vi "Main_ProductionMonitor.vi"() -> ()   [LabVIEW 2017]
uses:
  ScanPLC_Config.vi
panel:
  out "LineName":string
  in  "Cluster":cluster{"Goal":dbl}
  out "Shift":string
  out "Date/Time":string
  in  "stop":bool
  in  "Tab":T1(tab)
  out "PLC Count Int":i32
  out "PLC Count Bool":bool
  in  "ProductionToCloud":bool
  out "ProductionBoard":T2={"StartHour"=[{"Hour"=5, "Minute"=0}, {"Hour"=6, "Minute"=0}, {"Hour"=7, "Minute"=0}, {"Hour"=7, "Minute"=30}, {"Hour"=0, "Minute"=0}, {"Hour"=0, "Minute"=0}, {"Hour"=0, "Minute"=0}, {"Hour"=0, "Minute"=0}, {"Hour"=0, "Minute"=0}], "Goal"=[], "EndHour"=[{"Hour"=5, "Minute"=59}, {"Hour"=6, "Minute"=59}, {"Hour"=7, "Minute"=10}, {"Hour"=7, "Minute"=59}, {"Hour"=0, "Minute"=0}, {"Hour"=0, "Minute"=0}, {"Hour"=0, "Minute"=0}, {"Hour"=0, "Minute"=0}, {"Hour"=0, "Minute"=0}], "AM/PM"=[{"AM/PM"=0}, {"AM/PM"=0}, {"AM/PM"=0}, {"AM/PM"=0}, {"AM/PM"=0}, {"AM/PM"=0}, {"AM/PM"=0}, {"AM/PM"=0}, {"AM/PM"=0}], "Actual"=[], "%"=[], "Status"=[], "Comments"=[]} {"AM/PM"."AM/PM" items=["AM", "PM"]; "EndHour"."Minute" items=["00", "1", "2", "3", "4", "5", "6", "7", "8", "9", "10", "11", "12", "13", "14", "15", "16", "17", "18", "19", "20", "21", "22", "23", "24", "25", "26", "27", "28", "29", "30", "31", "32", "33", "34", "35", "36", "37", "38", "39", "40", "41", "42", "43", "44", "45", "46", "47", "48", "49", "50", "51", "52", "53", "54", "55", "56", "57", "58", "59"]; "EndHour"."Hour" items=["00", "1", "2", "3", "4", "5", "6", "7", "8", "9", "10", "11", "12", "13", "14", "15", "16", "17", "18", "19", "20", "21", "22", "23"]; "StartHour"."Minute" items=["00", "1", "2", "3", "4", "5", "6", "7", "8", "9", "10", "11", "12", "13", "14", "15", "16", "17", "18", "19", "20", "21", "22", "23", "24", "25", "26", "27", "28", "29", "30", "31", "32", "33", "34", "35", "36", "37", "38", "39", "40", "41", "42", "43", "44", "45", "46", "47", "48", "49", "50", "51", "52", "53", "54", "55", "56", "57", "58", "59"]; "StartHour"."Hour" items=["00", "1", "2", "3", "4", "5", "6", "7", "8", "9", "10", "11", "12", "13", "14", "15", "16", "17", "18", "19", "20", "21", "22", "23"]}
  in  "ShiftsFromCloud":bool
  in  "ShiftsToCloud":bool
  in  "Refresh Button":bool
  in  "GoalCalc":bool
  in  "SaveShifts":bool
  in  "3rdShiftConfig":T3={"StartHour"=[{"Hour"=5, "Minute"=0}, {"Hour"=6, "Minute"=0}, {"Hour"=7, "Minute"=0}, {"Hour"=7, "Minute"=30}, {"Hour"=0, "Minute"=0}, {"Hour"=0, "Minute"=0}, {"Hour"=0, "Minute"=0}, {"Hour"=0, "Minute"=0}, {"Hour"=0, "Minute"=0}], "Goal"=[], "EndHour"=[{"Hour"=5, "Minute"=59}, {"Hour"=6, "Minute"=59}, {"Hour"=7, "Minute"=10}, {"Hour"=7, "Minute"=59}, {"Hour"=0, "Minute"=0}, {"Hour"=0, "Minute"=0}, {"Hour"=0, "Minute"=0}, {"Hour"=0, "Minute"=0}, {"Hour"=0, "Minute"=0}], "AM/PM"=[]} caption="3rdShift" {"AM/PM"."AM/PM" items=["AM", "PM"]; "EndHour"."Minute" items=["00", "1", "2", "3", "4", "5", "6", "7", "8", "9", "10", "11", "12", "13", "14", "15", "16", "17", "18", "19", "20", "21", "22", "23", "24", "25", "26", "27", "28", "29", "30", "31", "32", "33", "34", "35", "36", "37", "38", "39", "40", "41", "42", "43", "44", "45", "46", "47", "48", "49", "50", "51", "52", "53", "54", "55", "56", "57", "58", "59"]; "EndHour"."Hour" items=["0", "1", "2", "3", "4", "5", "6", "7", "8", "9", "10", "11", "12", "13", "14", "15", "16", "17", "18", "19", "20", "21", "22", "23"]; "StartHour"."Minute" items=["00", "1", "2", "3", "4", "5", "6", "7", "8", "9", "10", "11", "12", "13", "14", "15", "16", "17", "18", "19", "20", "21", "22", "23", "24", "25", "26", "27", "28", "29", "30", "31", "32", "33", "34", "35", "36", "37", "38", "39", "40", "41", "42", "43", "44", "45", "46", "47", "48", "49", "50", "51", "52", "53", "54", "55", "56", "57", "58", "59"]; "StartHour"."Hour" items=["0", "1", "2", "3", "4", "5", "6", "7", "8", "9", "10", "11", "12", "13", "14", "15", "16", "17", "18", "19", "20", "21", "22", "23"]}
  in  "2ndShiftConfig":T3={"StartHour"=[{"Hour"=5, "Minute"=0}, {"Hour"=6, "Minute"=0}, {"Hour"=7, "Minute"=0}, {"Hour"=7, "Minute"=30}, {"Hour"=0, "Minute"=0}, {"Hour"=0, "Minute"=0}, {"Hour"=0, "Minute"=0}, {"Hour"=0, "Minute"=0}, {"Hour"=0, "Minute"=0}], "Goal"=[], "EndHour"=[{"Hour"=5, "Minute"=59}, {"Hour"=6, "Minute"=59}, {"Hour"=7, "Minute"=10}, {"Hour"=7, "Minute"=59}, {"Hour"=0, "Minute"=0}, {"Hour"=0, "Minute"=0}, {"Hour"=0, "Minute"=0}, {"Hour"=0, "Minute"=0}, {"Hour"=0, "Minute"=0}], "AM/PM"=[{"AM/PM"=1}, {"AM/PM"=1}, {"AM/PM"=1}, {"AM/PM"=1}, {"AM/PM"=1}, {"AM/PM"=1}, {"AM/PM"=1}, {"AM/PM"=1}, {"AM/PM"=1}]} caption="2ndShift" {"AM/PM"."AM/PM" items=["AM", "PM"]; "EndHour"."Minute" items=["00", "1", "2", "3", "4", "5", "6", "7", "8", "9", "10", "11", "12", "13", "14", "15", "16", "17", "18", "19", "20", "21", "22", "23", "24", "25", "26", "27", "28", "29", "30", "31", "32", "33", "34", "35", "36", "37", "38", "39", "40", "41", "42", "43", "44", "45", "46", "47", "48", "49", "50", "51", "52", "53", "54", "55", "56", "57", "58", "59"]; "EndHour"."Hour" items=["00", "1", "2", "3", "4", "5", "6", "7", "8", "9", "10", "11", "12", "13", "14", "15", "16", "17", "18", "19", "20", "21", "22", "23"]; "StartHour"."Minute" items=["00", "1", "2", "3", "4", "5", "6", "7", "8", "9", "10", "11", "12", "13", "14", "15", "16", "17", "18", "19", "20", "21", "22", "23", "24", "25", "26", "27", "28", "29", "30", "31", "32", "33", "34", "35", "36", "37", "38", "39", "40", "41", "42", "43", "44", "45", "46", "47", "48", "49", "50", "51", "52", "53", "54", "55", "56", "57", "58", "59"]; "StartHour"."Hour" items=["0", "1", "2", "3", "4", "5", "6", "7", "8", "9", "10", "11", "12", "13", "14", "15", "16", "17", "18", "19", "20", "21", "22", "23"]}
  in  "1stShiftConfig":T3={"StartHour"=[{"Hour"=5, "Minute"=0}, {"Hour"=6, "Minute"=0}, {"Hour"=7, "Minute"=0}, {"Hour"=7, "Minute"=30}, {"Hour"=0, "Minute"=0}, {"Hour"=0, "Minute"=0}, {"Hour"=0, "Minute"=0}, {"Hour"=0, "Minute"=0}, {"Hour"=0, "Minute"=0}], "Goal"=[], "EndHour"=[{"Hour"=5, "Minute"=59}, {"Hour"=6, "Minute"=59}, {"Hour"=7, "Minute"=10}, {"Hour"=7, "Minute"=59}, {"Hour"=0, "Minute"=0}, {"Hour"=0, "Minute"=0}, {"Hour"=0, "Minute"=0}, {"Hour"=0, "Minute"=0}, {"Hour"=0, "Minute"=0}], "AM/PM"=[{"AM/PM"=0}, {"AM/PM"=0}, {"AM/PM"=0}, {"AM/PM"=0}, {"AM/PM"=0}, {"AM/PM"=0}, {"AM/PM"=0}, {"AM/PM"=0}, {"AM/PM"=0}]} caption="1stShift" {"AM/PM"."AM/PM" items=["AM", "PM"]; "EndHour"."Minute" items=["00", "1", "2", "3", "4", "5", "6", "7", "8", "9", "10", "11", "12", "13", "14", "15", "16", "17", "18", "19", "20", "21", "22", "23", "24", "25", "26", "27", "28", "29", "30", "31", "32", "33", "34", "35", "36", "37", "38", "39", "40", "41", "42", "43", "44", "45", "46", "47", "48", "49", "50", "51", "52", "53", "54", "55", "56", "57", "58", "59"]; "EndHour"."Hour" items=["0", "1", "2", "3", "4", "5", "6", "7", "8", "9", "10", "11", "12", "13", "14", "15", "16", "17", "18", "19", "20", "21", "22", "23"]; "StartHour"."Minute" items=["00", "1", "2", "3", "4", "5", "6", "7", "8", "9", "10", "11", "12", "13", "14", "15", "16", "17", "18", "19", "20", "21", "22", "23", "24", "25", "26", "27", "28", "29", "30", "31", "32", "33", "34", "35", "36", "37", "38", "39", "40", "41", "42", "43", "44", "45", "46", "47", "48", "49", "50", "51", "52", "53", "54", "55", "56", "57", "58", "59"]; "StartHour"."Hour" items=["0", "1", "2", "3", "4", "5", "6", "7", "8", "9", "10", "11", "12", "13", "14", "15", "16", "17", "18", "19", "20", "21", "22", "23"]}
  out "Parts/Hour":dbl
  in  "Cycle Time (s)":dbl=25.0
  in  "ShiftConfigPath":path
  in  "MainConfigFromCloud":bool
  in  "MainConfigBackup":bool
  in  "MainConfigPath":path
  in  "MainConfigurationArray":cluster{"Parameter":string, "Value":string}[](array[cluster])
  in  "SaveMailConfig":bool
  in  "RefreshMailConfig":bool
  out "NotificationMessage":string
  in  "Mail Button":bool
  in  "MainConfigToCloud":bool
  in  "PLC Connection Array":T4(array[cluster]) {"MemoryType" items=["CR (Control Relay)", "MR (Internal Auxiliary Relay)", "VB (Work Relay)", "LR (Latch Relay)", "B (Link Relay)", "R (Relay)", "DM (Data Memory)", "EM (Extended Data Memory)", "FM (File Register 1)", "ZF (FIle Register 2)", "W (Link Register)", "TM (Temporary Data Memory)", "Z (Index Register)", "T (Timer)", "TC (Timer (Counter Value))", "TS (Timer Set Value)", "C (Counter)", "CC (Counter (Counter Value))", "CS (Counter (Set Value))", "CTH (High Speed Counter)", "CTC (High Speed Counter Comparator (Set Value))", "AT (Digital Trimmer)", "CM (Control Memory)", "VM (Work Memory)"]; "PLC Type" items=["Keyence", "Allen Bradley", "Mitsubishi", "Panasonic", "Siemens"]}
  in  "PLCConfigPath":path
  in  "RefreshPLCConfig":bool
  in  "SavePLCConfig":bool
  # "Hourly Production Report"
  # "MachineName"
  # "PLC Address"
  # "PLC Type"
  # "Memory Type"
  # "MemoryNumber"
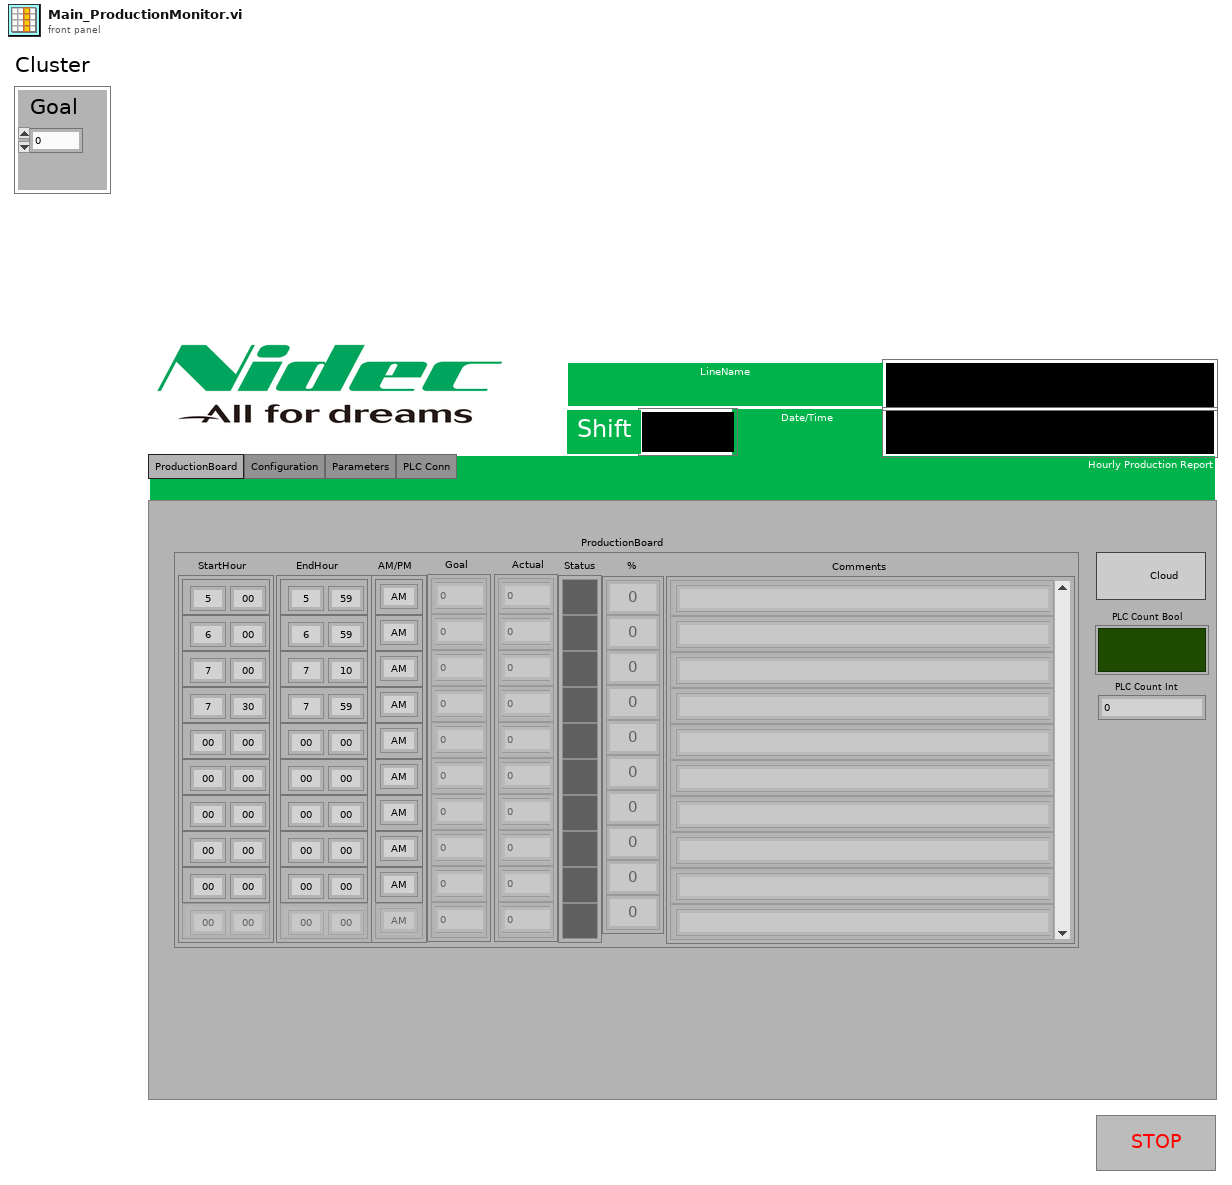
[diagram p1: front panel]
types:
  T1 = enum32{"ProductionBoard", "Configuration", "Parameters", "PLC Conn"}
  T2 = cluster{"StartHour":cluster{"Hour":u16, "Minute":u16}[], "Goal":cluster{"Goal":dbl}[], "EndHour":cluster{"Hour":u16, "Minute":u16}[], "AM/PM":cluster{"AM/PM":u16}[], "Actual":cluster{"Actual":dbl}[], "%":i32[], "Status":u32[], "Comments":cluster{"Comments":string}[]}
  T3 = cluster{"StartHour":cluster{"Hour":u16, "Minute":u16}[], "Goal":cluster{"Goal":dbl}[], "EndHour":cluster{"Hour":u16, "Minute":u16}[], "AM/PM":cluster{"AM/PM":u16}[]}
  T4 = cluster{"MachineName":string, "PLC Address":string, "PLC Type":u16, "MemoryType":u16, "MemoryNumber":i32}[]
  T5 = cluster{"MachineName":string, "PLC Address":string, "PLC Type":u16, "MemoryType":u16, "MemoryNumber":i32}
  T6 = cluster{"1stShiftConfig":cluster{"StartHour":cluster{"Hour":u16, "Minute":u16}[], "Goal":cluster{"Goal":dbl}[], "EndHour":cluster{"Hour":u16, "Minute":u16}[], "AM/PM":cluster{"AM/PM":u16}[]}, "2ndShiftConfig":cluster{"StartHour":cluster{"Hour":u16, "Minute":u16}[], "Goal":cluster{"Goal":dbl}[], "EndHour":cluster{"Hour":u16, "Minute":u16}[], "AM/PM":cluster{"AM/PM":u16}[]}, "3rdShiftConfig":cluster{"StartHour":cluster{"Hour":u16, "Minute":u16}[], "Goal":cluster{"Goal":dbl}[], "EndHour":cluster{"Hour":u16, "Minute":u16}[], "AM/PM":cluster{"AM/PM":u16}[]}}
  T7 = cluster{"Hour":cluster{"Hour":u16, "Minute":u16}}[]
  T8 = cluster{"InitialHour":u16, "InitialMinute":u16, "EndHour":u16, "EndMinute":u16, "Goal":dbl, "Actual":dbl, "Comments":string}[]
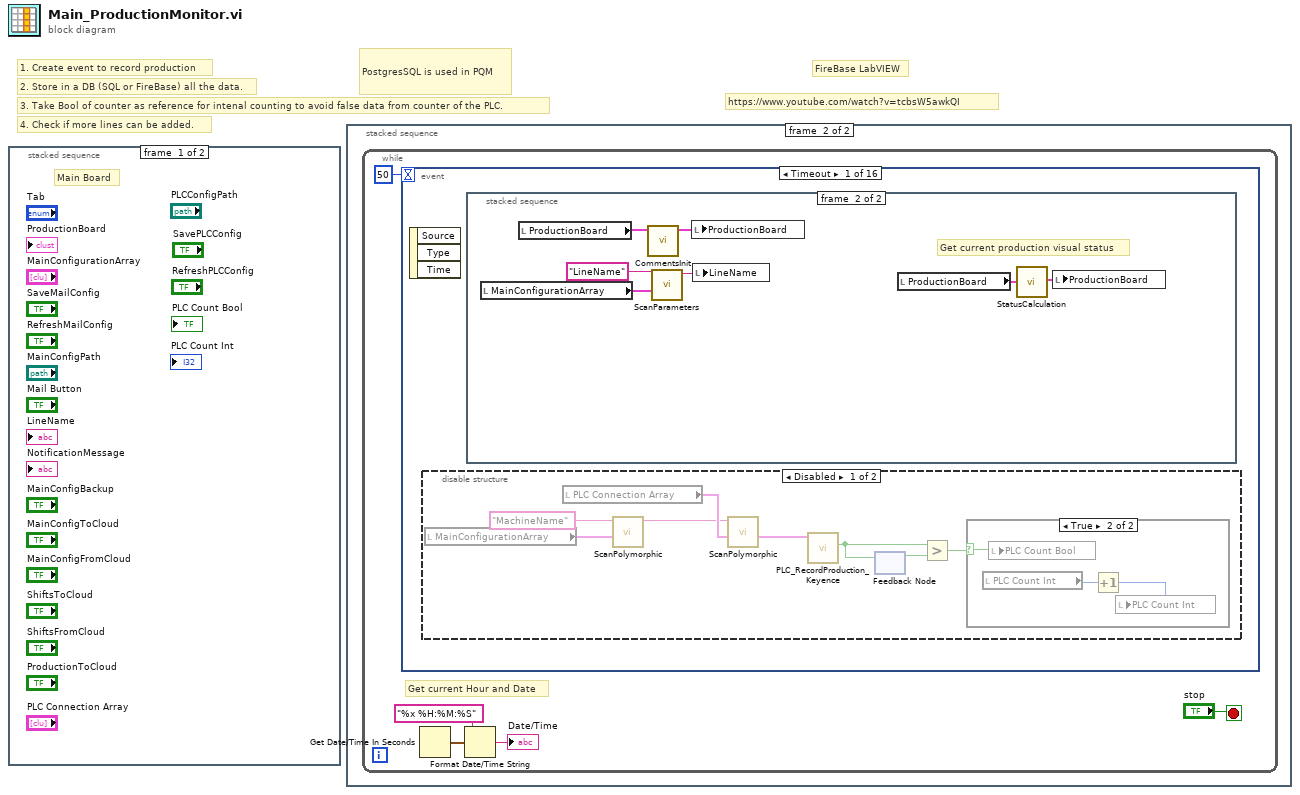
[diagram p0: block diagram]
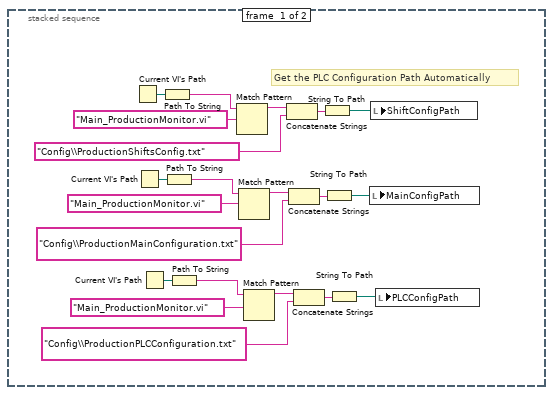
[diagram p2: hidden frame]
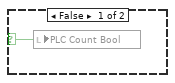
[diagram p3: hidden frame]
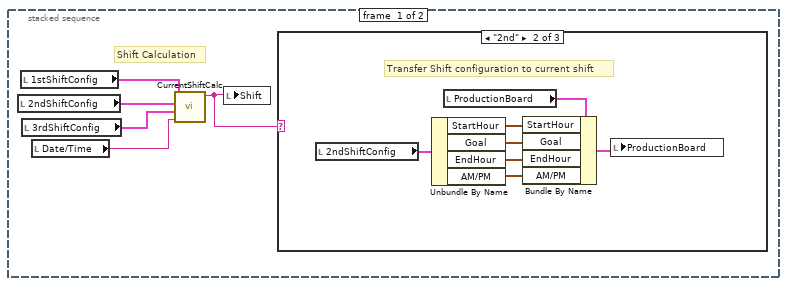
[diagram p5: hidden frame]
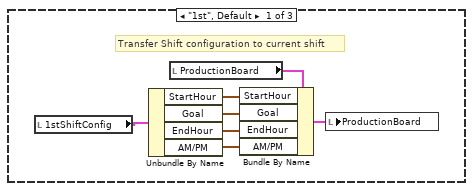
[diagram p6: hidden frame]
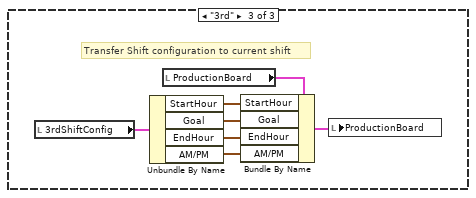
[diagram p7: hidden frame]
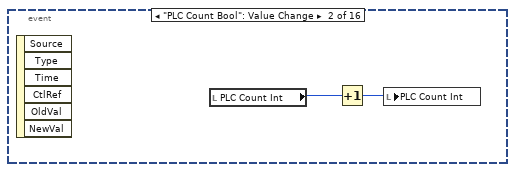
[diagram p8: hidden frame]
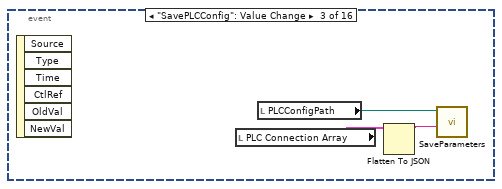
[diagram p9: hidden frame]
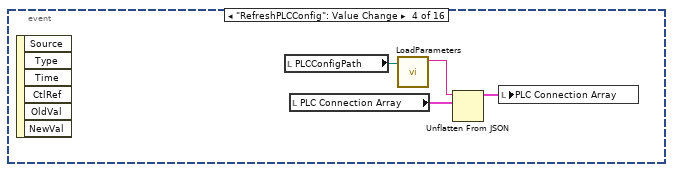
[diagram p10: hidden frame]
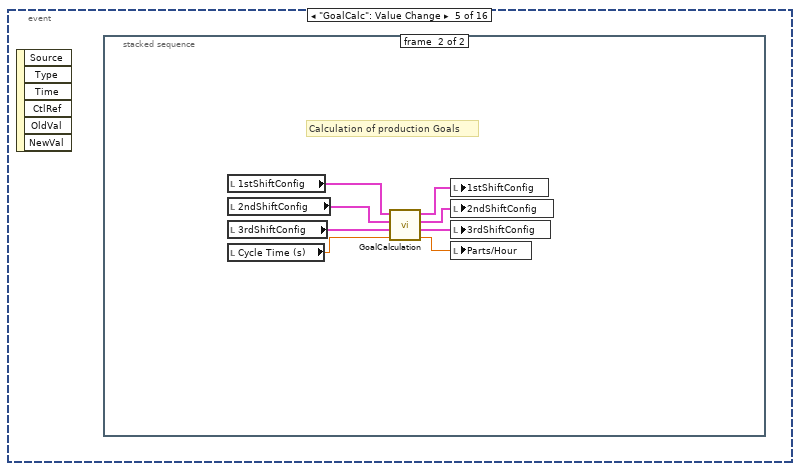
[diagram p11: hidden frame]
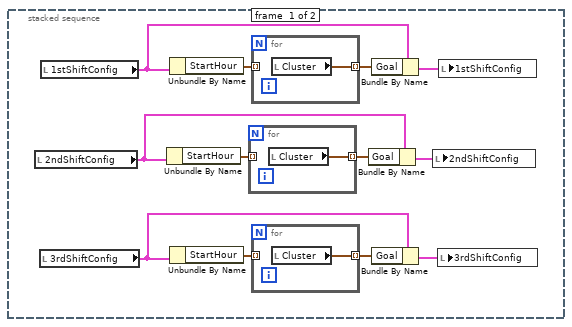
[diagram p12: hidden frame]
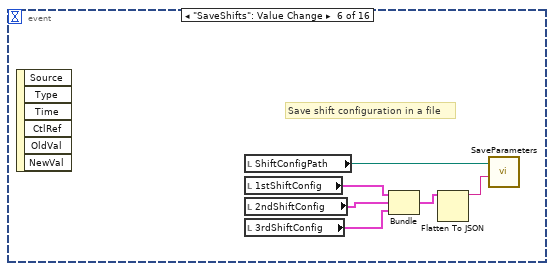
[diagram p13: hidden frame]
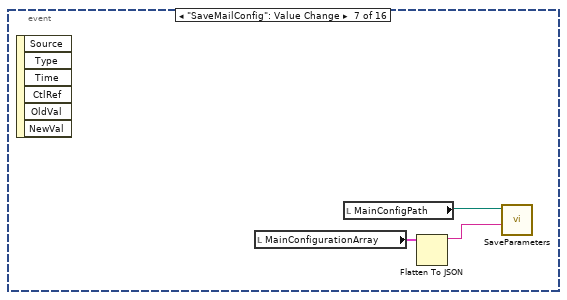
[diagram p14: hidden frame]
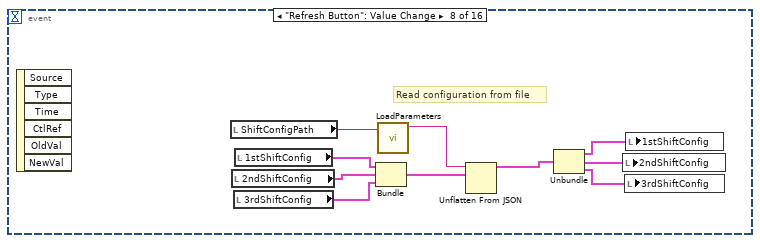
[diagram p15: hidden frame]
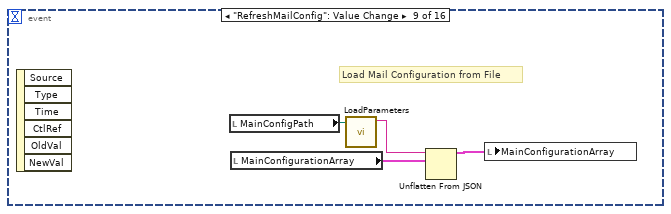
[diagram p16: hidden frame]
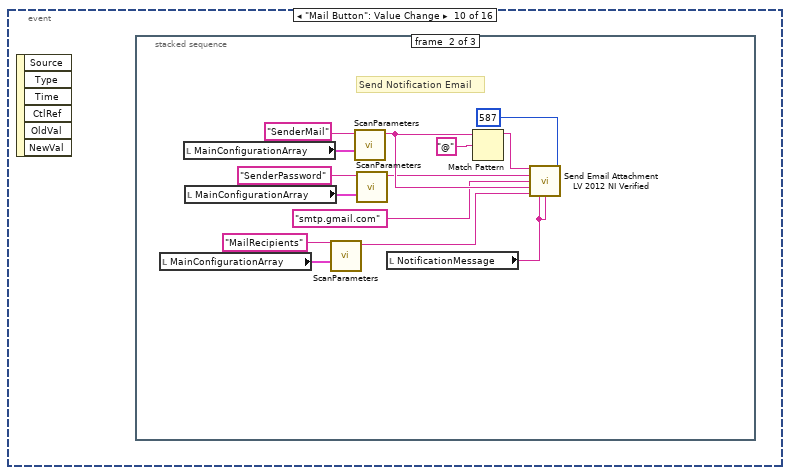
[diagram p17: hidden frame]
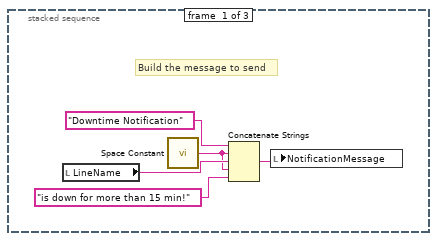
[diagram p18: hidden frame]
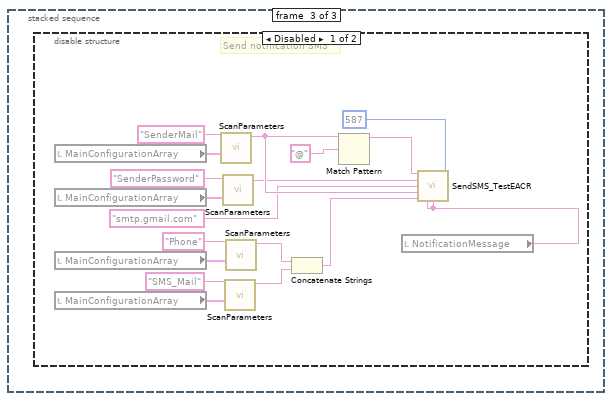
[diagram p19: hidden frame]
diagram:
  # "PostgresSQL is used in PQM"
  # "FireBase LabVIEW"
  # "https://www.youtube.com/watch?v=tcbsW5awkQI"
  # "4. Check if more lines can be added."
  # "2. Store in a DB (SQL or FireBase) all the data."
  # "1. Create event to record production"
  # "3. Take Bool of counter as reference for intenal counting to avoid false data from counter of the PLC."
  n1 = stacked-sequence {
    frame #0 {
      # "Main Board"
    }
    frame #1 {
      # "Configuration"
    }
  }
  n2 = stacked-sequence {
    frame #0 {
      # "Get the PLC Configuration Path Automatically"
      n3 = Current VI's Path() -> (path=w6:path)
      n4 = Current VI's Path() -> (path=w16:path)
      n5 = Current VI's Path() -> (path=w17:path)
      n6 = Path To String(path=w6) -> (string=w7:string)
      n7 = Path To String(path=w16) -> (string=w15:string)
      n8 = Path To String(path=w17) -> (string=w18:string)
      n9 = Match Pattern(string=w7, regular expression="Main_ProductionMonitor.vi") -> (before substring=w8:string)  [unwired: 1 in, 3 out]
      n10 = Match Pattern(string=w15, regular expression="Main_ProductionMonitor.vi") -> (before substring=w14:string)  [unwired: 1 in, 3 out]
      n11 = Match Pattern(string=w18, regular expression="Main_ProductionMonitor.vi") -> (before substring=w19:string)  [unwired: 1 in, 3 out]
      n12 = Concatenate Strings(w8, "Config\\ProductionShiftsConfig.txt" ("regular expression")) -> (w9:string)
      n13 = Concatenate Strings(w14, "Config\\ProductionMainConfiguration.txt" ("regular expression")) -> (w13:string)
      n14 = Concatenate Strings(w19, "Config\\ProductionPLCConfiguration.txt" ("regular expression")) -> (w20:string)
      n15 = String To Path(string=w9) -> (path=w3:path)
      n16 = String To Path(string=w13) -> (path=w2:path)
      n17 = String To Path(string=w20) -> (path=w1:path)
      n18 = local write "MainConfigPath"(w2) -> ()
      n19 = local write "ShiftConfigPath"(w3) -> ()
      n20 = local write "PLCConfigPath"(w1) -> ()
    }
    frame #1 {
      n21 = while {
        stop <- "stop" stop-if-true
        # "Get current Hour and Date"
        n22 = event shown="[0] Timeout" {
          selector: _ -> [_ _ _ _ _ _ _ _ _ _ _ _ _ _ _ _]
          dyn-events: _ -> [_ _ _ _ _ _ _ _ _ _ _ _ _ _ _ _]
          timeout: 50 -> [_ _ _ _ _ _ _ _ _ _ _ _ _ _ _ _]
          event Timeout {
            n23 = event-data() -> ()  [unwired: 1 in, 3 out]
            n24 = disable-structure shown="Disabled" {
              frame Disabled {
                n25 = local read "MainConfigurationArray"() -> (w34:cluster{"Parameter":string, "Value":string}[])
                n26 = local read "PLC Connection Array"() -> (w32:T4)
                n27 = call-poly "ScanPolymorphic.vi"("MainConfigurationArray"=w34, "Parameter"="MachineName") -> ("Value"=w31:string)  [unwired: 9 in]
                n28 = call-poly "ScanPolymorphic.vi"("PLC Connection Array"=w32, "Parameter"=w31) -> ("ConnectionInformation"=w30:T5)  [unwired: 9 in]
                n29 = call "PLC_RecordProduction_Keyence.vi"("ConnectionInformation"=w30) -> ("Bool State"=w27:bool)  [unwired: 10 in]
                n30 = feedback #1() -> (w29:bool)  [unwired: 1 in]
                n31 = feedback-in #1(w27) -> ()
                n32 = Greater?(x=w27, y=w29) -> (0:w28:bool)
                n33 = case shown="True" w28 {
                  selector: w28 -> [w35 w38]
                  frame False {
                    n34 = local write "PLC Count Bool"(w35) -> ()
                  }
                  frame True {
                    n35 = local read "PLC Count Int"() -> (w36:i32)
                    n36 = local write "PLC Count Bool"(w38) -> ()
                    n37 = Increment(x=w36) -> (x+1=w37:i32)
                    n38 = local write "PLC Count Int"(w37) -> ()
                  }
                }
              }
              frame Enabled {
              }
            }
            n39 = stacked-sequence {
              frame #0 {
                # "Shift Calculation"
                n40 = local read "2ndShiftConfig"() -> (w40:T3)
                n41 = local read "1stShiftConfig"() -> (w41:T3)
                n42 = local read "3rdShiftConfig"() -> (w39:T3)
                n43 = local read "Date/Time"() -> (w43:string)
                n44 = call "CurrentShiftCalc.vi"("Date/Time"=w43, "3rdShiftConfig"=w39, "2ndShiftConfig"=w40, "1stShiftConfig"=w41) -> ("Shift"=w42:string)  [unwired: 7 in]
                n45 = local write "Shift"(w42) -> ()
                n46 = case shown="\"2nd\"" w42 {
                  frame "1st", Default {
                    # "Transfer Shift configuration to current shift"
                    n47 = local read "1stShiftConfig"() -> (w50:T3)
                    n48 = Unbundle By Name(w50) -> ("StartHour"=w47:cluster{"Hour":u16, "Minute":u16}[], "Goal"=w46:cluster{"Goal":dbl}[], "EndHour"=w45:cluster{"Hour":u16, "Minute":u16}[], "AM/PM"=w44:cluster{"AM/PM":u16}[])
                    n49 = local read "ProductionBoard"() -> (w49:T2)
                    n50 = Bundle By Name(cluster=w49, "StartHour"=w47, "Goal"=w46, "EndHour"=w45, "AM/PM"=w44) -> (w48:T2)
                    n51 = local write "ProductionBoard"(w48) -> ()
                  }
                  frame "2nd" {
                    # "Transfer Shift configuration to current shift"
                    n52 = local read "2ndShiftConfig"() -> (w57:T3)
                    n53 = Unbundle By Name(w57) -> ("StartHour"=w54:cluster{"Hour":u16, "Minute":u16}[], "Goal"=w53:cluster{"Goal":dbl}[], "EndHour"=w52:cluster{"Hour":u16, "Minute":u16}[], "AM/PM"=w51:cluster{"AM/PM":u16}[])
                    n54 = local read "ProductionBoard"() -> (w56:T2)
                    n55 = Bundle By Name(cluster=w56, "StartHour"=w54, "Goal"=w53, "EndHour"=w52, "AM/PM"=w51) -> (w55:T2)
                    n56 = local write "ProductionBoard"(w55) -> ()
                  }
                  frame "3rd" {
                    # "Transfer Shift configuration to current shift"
                    n57 = local read "3rdShiftConfig"() -> (w64:T3)
                    n58 = Unbundle By Name(w64) -> ("StartHour"=w61:cluster{"Hour":u16, "Minute":u16}[], "Goal"=w60:cluster{"Goal":dbl}[], "EndHour"=w59:cluster{"Hour":u16, "Minute":u16}[], "AM/PM"=w58:cluster{"AM/PM":u16}[])
                    n59 = local read "ProductionBoard"() -> (w63:T2)
                    n60 = Bundle By Name(cluster=w63, "StartHour"=w61, "Goal"=w60, "EndHour"=w59, "AM/PM"=w58) -> (w62:T2)
                    n61 = local write "ProductionBoard"(w62) -> ()
                  }
                }
              }
              frame #1 {
                # "Get current production visual status"
                n62 = local read "MainConfigurationArray"() -> (w68:cluster{"Parameter":string, "Value":string}[])
                n63 = local read "ProductionBoard"() -> (w71:T2)
                n64 = call "CommentsInit.vi"("ProductionBoardIN"=w71) -> ("ProductionBoardOUT"=w70:T2)  [unwired: 10 in]
                n65 = call "ScanParameters.vi"("MainConfigurationArray"=w68, "Parameter"="LineName") -> ("Value"=w69:string)  [unwired: 9 in]
                n66 = local write "ProductionBoard"(w70) -> ()
                n67 = local write "LineName"(w69) -> ()
                n68 = local read "ProductionBoard"() -> (w65:T2)
                n69 = call "StatusCalculation.vi"("ProductionBoard"=w65) -> ("ProductionBoard 2"=w66:T2)
                n70 = local write "ProductionBoard"(w66) -> ()
              }
            }
          }
          event "PLC Count Bool": Value Change {
            n71 = event-data() -> ()  [unwired: 1 in, 6 out]
            n72 = local read "PLC Count Int"() -> (w73:i32)
            n73 = Increment(x=w73) -> (x+1=w72:i32)
            n74 = local write "PLC Count Int"(w72) -> ()
          }
          event "SavePLCConfig": Value Change {
            n75 = event-data() -> ()  [unwired: 1 in, 6 out]
            n76 = local read "PLC Connection Array"() -> (w75:T4)
            n77 = local read "PLCConfigPath"() -> (w76:path)
            n78 = Flatten To JSON(anything=w75) -> (JSON string=w74:string)  [unwired: 2 in, 1 out]
            n79 = call "SaveParameters.vi"("JSON_Text"=w74, "ShiftConfigPath"=w76) -> ()  [unwired: 10 in]
          }
          event "RefreshPLCConfig": Value Change {
            n80 = event-data() -> ()  [unwired: 1 in, 6 out]
            n81 = local read "PLCConfigPath"() -> (w80:path)
            n82 = local read "PLC Connection Array"() -> (w79:T4)
            n83 = call "LoadParameters.vi"("ShiftConfigPath"=w80) -> ("JSON_Text"=w78:string)  [unwired: 10 in]
            n84 = Unflatten From JSON(JSON string=w78, type and defaults=w79) -> (value=w77:T4)  [unwired: 5 in, 1 out]
            n85 = local write "PLC Connection Array"(w77) -> ()
          }
          event "GoalCalc": Value Change {
            n86 = event-data() -> ()  [unwired: 1 in, 6 out]
            n87 = stacked-sequence {
              frame #0 {
                n88 = local read "2ndShiftConfig"() -> (w86:T3)
                n89 = local read "3rdShiftConfig"() -> (w83:T3)
                n90 = local read "1stShiftConfig"() -> (w91:T3)
                n91 = Unbundle By Name(w86) -> ("StartHour"=w87:cluster{"Hour":u16, "Minute":u16}[])
                n92 = Unbundle By Name(w91) -> ("StartHour"=w90:cluster{"Hour":u16, "Minute":u16}[])
                n93 = Unbundle By Name(w83) -> ("StartHour"=w82:cluster{"Hour":u16, "Minute":u16}[])
                n94 = for {
                  tunnel: w87 -> [_] mode=indexing
                  tunnel: [w94] -> w88 mode=indexing
                  n95 = local read "Cluster"() -> (w94:cluster{"Goal":dbl})
                }
                n96 = for {
                  tunnel: w90 -> [_] mode=indexing
                  tunnel: [w95] -> w89 mode=indexing
                  n97 = local read "Cluster"() -> (w95:cluster{"Goal":dbl})
                }
                n98 = for {
                  tunnel: w82 -> [_] mode=indexing
                  tunnel: [w93] -> w81 mode=indexing
                  n99 = local read "Cluster"() -> (w93:cluster{"Goal":dbl})
                }
                n100 = Bundle By Name(cluster=w86, "Goal"=w88) -> (w85:T3)
                n101 = Bundle By Name(cluster=w91, "Goal"=w89) -> (w92:T3)
                n102 = Bundle By Name(cluster=w83, "Goal"=w81) -> (w84:T3)
                n103 = local write "2ndShiftConfig"(w85) -> ()
                n104 = local write "3rdShiftConfig"(w84) -> ()
                n105 = local write "1stShiftConfig"(w92) -> ()
              }
              frame #1 {
                # "Calculation of production Goals"
                n106 = local read "1stShiftConfig"() -> (w103:T3)
                n107 = local read "2ndShiftConfig"() -> (w102:T3)
                n108 = local read "3rdShiftConfig"() -> (w101:T3)
                n109 = local read "Cycle Time (s)"() -> (w100:dbl)
                n110 = call "GoalCalculation.vi"("CycleTimeInput"=w100, "3rdShiftConfig"=w101, "2ndShiftConfig"=w102, "1stShiftConfig"=w103) -> ("Parts/Hour"=w96:dbl, "3rdShiftConfig 2"=w97:T3, "2ndShiftConfig 2"=w98:T3, "1stShiftConfig 2"=w99:T3)  [unwired: 3 in]
                n111 = local write "1stShiftConfig"(w99) -> ()
                n112 = local write "2ndShiftConfig"(w98) -> ()
                n113 = local write "3rdShiftConfig"(w97) -> ()
                n114 = local write "Parts/Hour"(w96) -> ()
              }
            }
          }
          event "SaveShifts": Value Change {
            # "Save shift configuration in a file"
            n115 = event-data() -> ()  [unwired: 1 in, 6 out]
            n116 = local read "ShiftConfigPath"() -> (w104:path)
            n117 = local read "1stShiftConfig"() -> (w108:T3)
            n118 = local read "2ndShiftConfig"() -> (w106:T3)
            n119 = local read "3rdShiftConfig"() -> (w109:T3)
            n120 = Bundle("1stShiftConfig"=w108, "2ndShiftConfig"=w106, "3rdShiftConfig"=w109) -> (w107:T6)  [unwired: 1 in]
            n121 = Flatten To JSON(anything=w107) -> (JSON string=w105:string)  [unwired: 2 in, 1 out]
            n122 = call "SaveParameters.vi"("JSON_Text"=w105, "ShiftConfigPath"=w104) -> ()  [unwired: 10 in]
          }
          event "SaveMailConfig": Value Change {
            n123 = event-data() -> ()  [unwired: 1 in, 6 out]
            n124 = local read "MainConfigurationArray"() -> (w112:cluster{"Parameter":string, "Value":string}[])
            n125 = local read "MainConfigPath"() -> (w110:path)
            n126 = Flatten To JSON(anything=w112) -> (JSON string=w111:string)  [unwired: 2 in, 1 out]
            n127 = call "SaveParameters.vi"("JSON_Text"=w111, "ShiftConfigPath"=w110) -> ()  [unwired: 10 in]
          }
          event "Refresh Button": Value Change {
            # "Read configuration from file"
            n128 = event-data() -> ()  [unwired: 1 in, 6 out]
            n129 = local read "ShiftConfigPath"() -> (w113:path)
            n130 = local read "2ndShiftConfig"() -> (w121:T3)
            n131 = local read "3rdShiftConfig"() -> (w122:T3)
            n132 = local read "1stShiftConfig"() -> (w120:T3)
            n133 = Bundle("1stShiftConfig"=w120, "2ndShiftConfig"=w121, "3rdShiftConfig"=w122) -> (w119:T6)  [unwired: 1 in]
            n134 = call "LoadParameters.vi"("ShiftConfigPath"=w113) -> ("JSON_Text"=w114:string)  [unwired: 10 in]
            n135 = Unflatten From JSON(JSON string=w114, type and defaults=w119) -> (value=w118:T6)  [unwired: 5 in, 1 out]
            n136 = Unbundle(w118) -> ("1stShiftConfig"=w117:T3, "2ndShiftConfig"=w116:T3, "3rdShiftConfig"=w115:T3)
            n137 = local write "2ndShiftConfig"(w116) -> ()
            n138 = local write "3rdShiftConfig"(w115) -> ()
            n139 = local write "1stShiftConfig"(w117) -> ()
          }
          event "RefreshMailConfig": Value Change {
            # "Load Mail Configuration from File"
            n140 = event-data() -> ()  [unwired: 1 in, 6 out]
            n141 = local read "MainConfigPath"() -> (w126:path)
            n142 = local read "MainConfigurationArray"() -> (w124:cluster{"Parameter":string, "Value":string}[])
            n143 = call "LoadParameters.vi"("ShiftConfigPath"=w126) -> ("JSON_Text"=w125:string)  [unwired: 10 in]
            n144 = Unflatten From JSON(JSON string=w125, type and defaults=w124) -> (value=w123:cluster{"Parameter":string, "Value":string}[])  [unwired: 5 in, 1 out]
            n145 = local write "MainConfigurationArray"(w123) -> ()
          }
          event "Mail Button": Value Change {
            n146 = event-data() -> ()  [unwired: 1 in, 6 out]
            n147 = stacked-sequence {
              frame #0 {
                # "Build the message to send"
                n148 = local read "LineName"() -> (w130:string)
                n149 = call <vilib>:"Space Constant.vi"() -> ("String"=w127:string)
                n150 = Concatenate Strings("Downtime Notification" ("Subject:"), w127, w130, w127, "is down for more than 15 min!" ("Subject:")) -> (w131:string)
                n151 = local write "NotificationMessage"(w131) -> ()
              }
              frame #1 {
                # "Send Notification Email"
                n152 = local read "MainConfigurationArray"() -> (w134:cluster{"Parameter":string, "Value":string}[])
                n153 = local read "MainConfigurationArray"() -> (w145:cluster{"Parameter":string, "Value":string}[])
                n154 = local read "MainConfigurationArray"() -> (w140:cluster{"Parameter":string, "Value":string}[])
                n155 = call "ScanParameters.vi"("MainConfigurationArray"=w134, "Parameter"="MailRecipients") -> ("Value"=w132:string)  [unwired: 9 in]
                n156 = call "ScanParameters.vi"("MainConfigurationArray"=w145, "Parameter"="SenderMail") -> ("Value"=w143:string)  [unwired: 9 in]
                n157 = call "ScanParameters.vi"("MainConfigurationArray"=w140, "Parameter"="SenderPassword") -> ("Value"=w138:string)  [unwired: 9 in]
                n158 = local read "NotificationMessage"() -> (w135:string)
                n159 = Match Pattern(string=w143, regular expression="@") -> (before substring=w141:string)  [unwired: 1 in, 3 out]
                n160 = call "Send Email Attachment LV 2012 NI Verified.vi"("Email Account ID"=w141, "Port"=587, "Email Account Password"=w138, "SMTP Outgoing Mail Server"="smtp.gmail.com" ("Parameter"), "From: (email@site.com)"=w143, "To: (email@site.com)"=w132, "Subject:"=w135, "Body:"=w135) -> ()  [unwired: 7 in, 1 out]
              }
              frame #2 {
                n161 = disable-structure shown="Disabled" {
                  frame Disabled {
                    # "Send notification SMS"
                    n162 = local read "MainConfigurationArray"() -> (w163:cluster{"Parameter":string, "Value":string}[])
                    n163 = local read "MainConfigurationArray"() -> (w162:cluster{"Parameter":string, "Value":string}[])
                    n164 = local read "MainConfigurationArray"() -> (w152:cluster{"Parameter":string, "Value":string}[])
                    n165 = local read "MainConfigurationArray"() -> (w151:cluster{"Parameter":string, "Value":string}[])
                    n166 = call "ScanParameters.vi"("MainConfigurationArray"=w163, "Parameter"="SenderMail") -> ("Value"=w157:string)  [unwired: 9 in]
                    n167 = call "ScanParameters.vi"("MainConfigurationArray"=w162, "Parameter"="SenderPassword") -> ("Value"=w155:string)  [unwired: 9 in]
                    n168 = call "ScanParameters.vi"("MainConfigurationArray"=w151, "Parameter"="SMS_Mail") -> ("Value"=w148:string)  [unwired: 9 in]
                    n169 = call "ScanParameters.vi"("MainConfigurationArray"=w152, "Parameter"="Phone") -> ("Value"=w149:string)  [unwired: 9 in]
                    n170 = Concatenate Strings(w149, w148) -> (w147:string)
                    n171 = Match Pattern(string=w157, regular expression="@") -> (before substring=w158:string)  [unwired: 1 in, 3 out]
                    n172 = local read "NotificationMessage"() -> (w156:string)
                    n173 = call "SendSMS_TestEACR.vi"("Email Account ID"=w158, "Port"=587, "Email Account Password"=w155, "SMTP Outgoing Mail Server"="smtp.gmail.com" ("Parameter"), "From: (email@site.com)"=w157, "To: (email@site.com)"=w147, "Subject:"=w156, "Body:"=w156) -> ()  [unwired: 7 in, 1 out]
                  }
                  frame Enabled {
                  }
                }
              }
            }
          }
          event "MainConfigBackup": Value Change {
            n174 = event-data() -> ()  [unwired: 1 in, 6 out]
            n175 = local read "MainConfigPath"() -> (w165:path)
            n176 = local read "ShiftConfigPath"() -> (w164:path)
            n177 = Path To String(path=w165) -> (string=w168:string)
            n178 = Not Equal?(x=w168, y="") -> (x != y?=w167:bool)
            n179 = case shown="True" w167 {
              tunnel: w165 -> [_ w175]
              tunnel: w164 -> [_ w174]
              frame False {
                n180 = One Button Dialog(message="No se eligio ningun archivo para respaldar") -> ()  [unwired: 1 in, 1 out]
              }
              frame True {
                n181 = Current VI's Path() -> (path=w173:path)
                n182 = call "ConfigFileBackup.vi"("CurrentVIPath"=w173, "ConfigFilePath"=w175) -> ("Success?"=w172:bool)  [unwired: 9 in]
                n183 = call "ConfigFileBackup.vi"("CurrentVIPath"=w173, "ConfigFilePath"=w174) -> ("Success?"=w171:bool)  [unwired: 9 in]
                n184 = And(x=w172, y=w171) -> (x .and. y?=w170:bool)
                n185 = case shown="True" w170 {
                  frame False {
                  }
                  frame True {
                    n186 = One Button Dialog(message="Backup Successful!") -> ()  [unwired: 1 in, 1 out]
                  }
                }
              }
            }
          }
          event "MainConfigToCloud": Value Change {
            n187 = event-data() -> ()  [unwired: 1 in, 6 out]
            n188 = local read "MainConfigurationArray"() -> (w179:cluster{"Parameter":string, "Value":string}[])
            n189 = local read "MainConfigurationArray"() -> (w180:cluster{"Parameter":string, "Value":string}[])
            n190 = call "ScanParameters.vi"("MainConfigurationArray"=w179, "Parameter"="CloudAddress") -> ("Value"=w177:string)  [unwired: 9 in]
            n191 = Flatten To JSON(anything=w180) -> (JSON string=w182:string)  [unwired: 2 in, 1 out]
            n192 = call "SaveDataInCloud.vi"("DataToBeStored"=w182, "FileName"="MainConfig.json", "CloudAddress"=w177) -> ()  [unwired: 9 in]
          }
          event "MainConfigFromCloud": Value Change {
            n193 = event-data() -> ()  [unwired: 1 in, 6 out]
            n194 = local read "MainConfigurationArray"() -> (w189:cluster{"Parameter":string, "Value":string}[])
            n195 = local read "MainConfigurationArray"() -> (w185:cluster{"Parameter":string, "Value":string}[])
            n196 = call "ScanParameters.vi"("MainConfigurationArray"=w189, "Parameter"="CloudAddress") -> ("Value"=w187:string)  [unwired: 9 in]
            n197 = call "LoadDataFromCloud.vi"("FileName"="MainConfig.json", "CloudAddress"=w187) -> ("DataReadFromCloud(json)"=w184:string)  [unwired: 9 in]
            n198 = Unflatten From JSON(JSON string=w184, type and defaults=w185) -> (value=w183:cluster{"Parameter":string, "Value":string}[])  [unwired: 5 in, 1 out]
            n199 = local write "MainConfigurationArray"(w183) -> ()
          }
          event "ShiftsFromCloud": Value Change {
            n200 = event-data() -> ()  [unwired: 1 in, 6 out]
            n201 = local read "MainConfigurationArray"() -> (w210:cluster{"Parameter":string, "Value":string}[])
            n202 = local read "MainConfigurationArray"() -> (w197:cluster{"Parameter":string, "Value":string}[])
            n203 = local read "MainConfigurationArray"() -> (w196:cluster{"Parameter":string, "Value":string}[])
            n204 = local read "2ndShiftConfig"() -> (w208:T3)
            n205 = local read "1stShiftConfig"() -> (w199:T3)
            n206 = local read "3rdShiftConfig"() -> (w194:T3)
            n207 = call "ScanParameters.vi"("MainConfigurationArray"=w210, "Parameter"="CloudAddress") -> ("Value"=w209:string)  [unwired: 9 in]
            n208 = call "ScanParameters.vi"("MainConfigurationArray"=w197, "Parameter"="CloudAddress") -> ("Value"=w198:string)  [unwired: 9 in]
            n209 = call "ScanParameters.vi"("MainConfigurationArray"=w196, "Parameter"="CloudAddress") -> ("Value"=w195:string)  [unwired: 9 in]
            n210 = call "LoadDataFromCloud.vi"("FileName"="2ndShiftConfig.json", "CloudAddress"=w209) -> ("DataReadFromCloud(json)"=w207:string)  [unwired: 9 in]
            n211 = call "LoadDataFromCloud.vi"("FileName"="1stShiftConfig.json", "CloudAddress"=w198) -> ("DataReadFromCloud(json)"=w200:string)  [unwired: 9 in]
            n212 = call "LoadDataFromCloud.vi"("FileName"="3rdShiftConfig.json", "CloudAddress"=w195) -> ("DataReadFromCloud(json)"=w193:string)  [unwired: 9 in]
            n213 = Unflatten From JSON(JSON string=w207, type and defaults=w208) -> (value=w206:T3)  [unwired: 5 in, 1 out]
            n214 = Unflatten From JSON(JSON string=w200, type and defaults=w199) -> (value=w201:T3)  [unwired: 5 in, 1 out]
            n215 = Unflatten From JSON(JSON string=w193, type and defaults=w194) -> (value=w192:T3)  [unwired: 5 in, 1 out]
            n216 = local write "2ndShiftConfig"(w206) -> ()
            n217 = local write "1stShiftConfig"(w201) -> ()
            n218 = local write "3rdShiftConfig"(w192) -> ()
          }
          event "ShiftsToCloud": Value Change {
            w215 = 0
            n219 = event-data() -> ()  [unwired: 1 in, 6 out]
            n220 = local read "1stShiftConfig"() -> (w218:T3)
            n221 = local read "1stShiftConfig"() -> (w217:T3)
            n222 = local read "MainConfigurationArray"() -> (w222:cluster{"Parameter":string, "Value":string}[])
            n223 = Unbundle By Name(w218) -> ("StartHour"=w216:cluster{"Hour":u16, "Minute":u16}[])
            n224 = Unbundle By Name(w217) -> ("EndHour"=w214:cluster{"Hour":u16, "Minute":u16}[])
            n225 = Index Array(array=w216, index=w215) -> (element=w212:cluster{"Hour":u16, "Minute":u16})
            n226 = Index Array(array=w214, index=w215) -> (element=w213:cluster{"Hour":u16, "Minute":u16})
            n227 = call "ScanParameters.vi"("MainConfigurationArray"=w222, "Parameter"="CloudAddress") -> ("Value"=w221:string)  [unwired: 9 in]
            n228 = Build Cluster Array(w212, w213) -> (w211:T7)
            n229 = Flatten To JSON(anything=w211) -> (JSON string=w223:string)  [unwired: 2 in, 1 out]
            n230 = call "SaveDataInCloud.vi"("DataToBeStored"=w223, "FileName"="1stShiftConfig.json", "CloudAddress"=w221) -> ()  [unwired: 9 in]
          }
          event "ProductionToCloud": Value Change {
            w229 = "_"
            # "ProductionBoard_011222_2nd.json"
            n231 = event-data() -> ()  [unwired: 1 in, 6 out]
            n232 = local read "ProductionBoard"() -> (w237:T2)
            n233 = Get Date/Time In Seconds() -> (seconds since 1Jan1904=w231:timestamp)
            n234 = local read "MainConfigurationArray"() -> (w235:cluster{"Parameter":string, "Value":string}[])
            n235 = local read "Shift"() -> (w224:string)
            n236 = Format Date/Time String(time format string (%c)="%m%d%y", seconds (now)=w231) -> (date/time string=w228:string)  [unwired: 1 in]
            n237 = call "ProductionBoardReduction.vi"("ProductionBoard"=w237) -> ("CloudProductionBoard"=w225:T8)  [unwired: 10 in]
            n238 = call "ScanParameters.vi"("MainConfigurationArray"=w235, "Parameter"="CloudAddress") -> ("Value"=w234:string)  [unwired: 9 in]
            n239 = Flatten To JSON(anything=w225) -> (JSON string=w236:string)  [unwired: 2 in, 1 out]
            n240 = Concatenate Strings("ProductionBoard" ("Parameter"), w229, w228, w229, w224, ".json" ("FileName")) -> (w226:string)
            n241 = call "SaveDataInCloud.vi"("DataToBeStored"=w236, "FileName"=w226, "CloudAddress"=w234) -> ()  [unwired: 9 in]
          }
        }
        n242 = Get Date/Time In Seconds() -> (seconds since 1Jan1904=w25:timestamp)
        n243 = Format Date/Time String(time format string (%c)="%x %H:%M:%S", seconds (now)=w25) -> (date/time string=→"Date/Time":string)  [unwired: 1 in]
      }
    }
  }
